vi "ROI entry-User ROI event-Apply new ROI.vi"(8 "error in (no error)":errorcluster, 10 "Input cluster":T1 {"ROIs Info []"."Zoom" min=1.0 max=10.0 step=0.10000000149011612; "Last Image Display Event info"."Tool" items=["None", "Selection Tool", "Point Tool", "Line Tool", "Rectangle Tool", "Oval Tool", "Polygon Tool", "ClosedFreehandTool", "Annulus Tool", "Rotated Rectangle Tool", "Zoom Tool", "Pan Tool", "Polyline Tool", "Freehand Tool"]; "Last Image Display Event info"."Type" items=["No Event"=0, "Click Event"=1, "Draw Event"=2, "Size Event"=4, "Scroll Event"=5, "Double Click Event"=8]}) -> (0 "error IO":errorcluster)   [LabVIEW 2013]
uses:
  Typedefs/ROI Entry screen VI interface 1.ctl
  Typedefs/Last Image Display Event info.ctl
  Typedefs/ROI spec.ctl
  Typedefs/ROI ID Enum.ctl
  ROI Entry screen/Globals/gl_ROI Entry UI globals.vi
panel:
  out "Last valid":T1 {"ROIs Info []"."Zoom" min=1.0 max=10.0 step=0.10000000149011612; "Last Image Display Event info"."Tool" items=["None", "Selection Tool", "Point Tool", "Line Tool", "Rectangle Tool", "Oval Tool", "Polygon Tool", "ClosedFreehandTool", "Annulus Tool", "Rotated Rectangle Tool", "Zoom Tool", "Pan Tool", "Polyline Tool", "Freehand Tool"]; "Last Image Display Event info"."Type" items=["No Event"=0, "Click Event"=1, "Draw Event"=2, "Size Event"=4, "Scroll Event"=5, "Double Click Event"=8]}
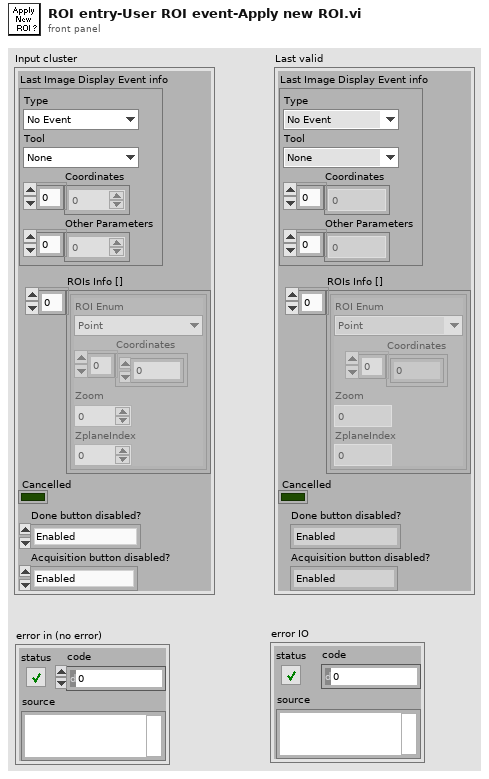
[diagram p1: front panel]
types:
  T1 = typedef "ROI Entry screen VI interface 1.ctl" = cluster{"Last Image Display Event info":T2, "ROIs Info []":T3[], "Cancelled":bool, "Done button disabled?":enum8{"Enabled", "Disabled", "Disabled and Grayed Out"}, "Acquisition button disabled?":enum8{"Enabled", "Disabled", "Disabled and Grayed Out"}}
  T2 = typedef "Last Image Display Event info.ctl" = cluster{"Type":i32, "Tool":i32, "Coordinates":i32[], "Other Parameters":sgl[]}
  T3 = typedef "ROI spec.ctl" = cluster{"Coordinates":i32[], "Zoom":dbl, "ROI Enum":T4, "ZplaneIndex":i32}
  T4 = typedef "ROI ID Enum.ctl" = enum16{"Point", "MiniScan", "Comp. MiniScan", "Rectangle", "Comp. volume", "Arb. plane point"}
  T5 = typedef "ROI entry screen ctrl refs cluster.ctl" = cluster{"Done button":refnum<vi>, "Imaging button":refnum<vi>, "Acquisition button":refnum<vi>, "POI dwell time (us)":refnum<vi>, "Scan dwell time per pixel (us)":refnum<vi>, "# of planes":refnum<vi>, "Zoom":refnum<vi>, "Equal size":refnum<vi>, "Channel":refnum<vi>, "Image Display":refnum<vi>, "Z-Plane Selector":refnum<vi>, "Number of lines left":refnum<vi>, "Z-stack folder path":refnum<vi>, "POI Density":refnum<vi>, "Arb Plane Entry":refnum<vi>, "Whole plane":refnum<vi>, "Clear Last":refnum<vi>, "Clear All":refnum<vi>, "Trial Length (sec)":refnum<vi>, "Palette Type":refnum<vi>, "Intensity slider":refnum<vi>, "# POI":refnum<vi>, "Max Z Proj":refnum<vi>, "Zplane ind":refnum<vi>, "Wavelength (nm)":refnum<vi>, "Number of Trials":refnum<vi>, "Funct stim.trig.enable":refnum<vi>, "Funct stim.trig.delay (s)":refnum<vi>, "Line Mode":refnum<vi>, "Step size (µm)":refnum<vi>, "ROI move mode":refnum<vi>, "Cool-down time (s)":refnum<vi>, "Enable cool-down time":refnum<vi>, "Motor Z ind. (um)":refnum<vi>, "AOL Z ind. (um)":refnum<vi>}
  T6 = enum8{"Enabled", "Disabled", "Disabled and Grayed Out"}
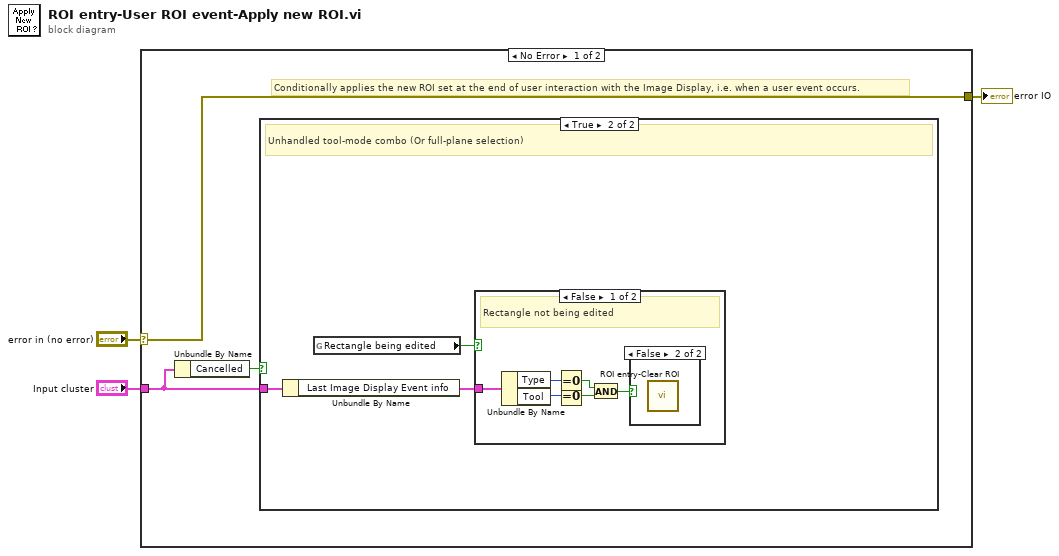
[diagram p0: block diagram]
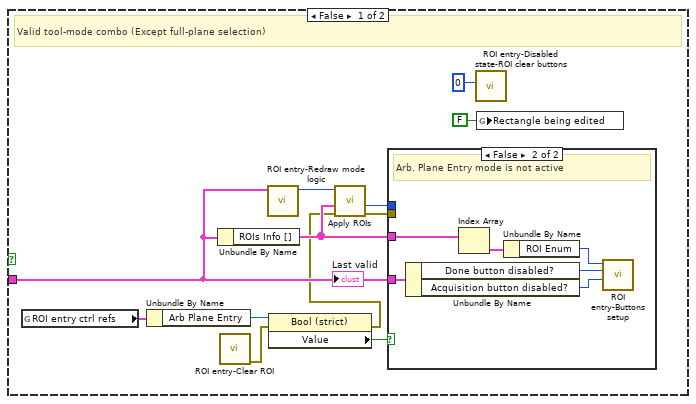
[diagram p2: hidden frame]
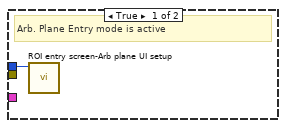
[diagram p3: hidden frame]
diagram:
  n1 = case shown="No Error" "error in (no error)" {
    selector: "error in (no error)" -> [w4 w35]
    tunnel: "Input cluster" -> [w6 _]
    tunnel: [w4 w35] -> w1
    frame No Error {
      # "Conditionally applies the new ROI set at the end of user interaction with the Image Display, i.e. when a user event occurs."
      n2 = Unbundle By Name(w6) -> ("Cancelled"=w5:bool)
      n3 = case shown="True" w5 {
        tunnel: w6 -> [w11 w27]
        frame False {
          # "Valid tool-mode combo (Except full-plane selection)"
          n4 = global read "gl_ROI Entry UI globals.vi" "ROI entry ctrl refs"() -> (w15:T5)
          n5 = Unbundle By Name(w15) -> ("Arb Plane Entry"=w16:refnum<vi>)
          n6 = Unbundle By Name(w11) -> ("ROIs Info []"=w12:T3[])
          n7 = call "ROI entry-Clear ROI.vi"() -> ("error out"=w9:errorcluster)  [unwired: 11 in]
          n8 = call "ROI entry-Redraw mode logic.vi"("Input cluster"=w11) -> ("Mode"=w13:enum16{"Redraw All", "Draw Last"})  [unwired: 10 in]
          n9 = property class="Bool (strict)"(reference=w16, error in=w9) -> (error out=w10:errorcluster, "Value"=w14:bool)  [unwired: 1 out]
          n10 = call "Apply ROIs.vi"("Mode (Redraw All)"=w13, "error in (no error)"=w10, "ROIs Info []"=w12) -> ("error out"=w17:errorcluster, "Number of ROI"=w18:i32)  [unwired: 5 in, 2 out]
          n11 = case shown="False" w14 {
            tunnel: w12 -> [_ w25]
            tunnel: w18 -> [w19 _]
            tunnel: w17 -> [_ _]
            tunnel: w11 -> [_ w22]
            frame True {
              # "Arb. Plane Entry mode is active"
              n12 = call "ROI entry screen-Arb plane UI setup.vi"("Number of ROI"=w19) -> ()  [unwired: 11 in]
            }
            frame False {
              # "Arb. Plane Entry mode is not active"
              n13 = Unbundle By Name(w22) -> ("Done button disabled?"=w21:T6, "Acquisition button disabled?"=w20:T6)
              n14 = Index Array(array=w25) -> (element=w24:T3)  [unwired: 1 in]
              n15 = Unbundle By Name(w24) -> ("ROI Enum"=w23:T4)
              n16 = call "ROI entry-Buttons setup.vi"("Acquisition button disabled?"=w20, "Done button disabled?"=w21, "ROI Enum"=w23) -> ()  [unwired: 9 in]
            }
          }
          n17 = call "ROI entry-Disabled state-ROI clear buttons.vi"("State"=0) -> ()  [unwired: 10 in, 1 out]
          n18 = global write "gl_ROI Entry UI globals.vi" "Rectangle being edited"(FALSE ("Rectangle being edited")) -> ()
          "Last valid" <- w11
        }
        frame True {
          # "Unhandled tool-mode combo (Or full-plane selection)"
          n19 = Unbundle By Name(w27) -> ("Last Image Display Event info"=w26:T2)
          n20 = global read "gl_ROI Entry UI globals.vi" "Rectangle being edited"() -> (w28:bool)
          n21 = case shown="False" w28 {
            tunnel: w26 -> [w31 _]
            frame False {
              # "Rectangle not being edited"
              n22 = Unbundle By Name(w31) -> ("Type"=w30:i32, "Tool"=w29:i32)
              n23 = Equal To 0?(x=w30) -> (x = 0?=w34:bool)
              n24 = Equal To 0?(x=w29) -> (x = 0?=w33:bool)
              n25 = And(x=w34, y=w33) -> (x .and. y?=w32:bool)
              n26 = case shown="False" w32 {
                frame True {
                }
                frame False {
                  n27 = call "ROI entry-Clear ROI.vi"() -> ()  [unwired: 11 in, 1 out]
                }
              }
            }
            frame True {
              # "Retains the NI ROI box\nto allow the user rotate it/edit it\nbefore accepting it."
              # "Rectangle being edited"
            }
          }
        }
      }
    }
    frame Error {
    }
  }
  "error IO" <- w1
